vi "GetLastLogFile.vi"(8 "error in (no error)":errorcluster) -> (0 "error out":errorcluster, 2 "Last log file name":string, 3 "Last log file path":path)   [LabVIEW 2013, in "ErrorMessage.lvclass"]
uses:
  001 - MAIN/Class/Messages/ErrorMessage/ErrorMessage.lvclass
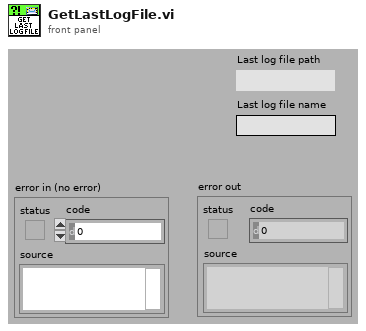
[diagram p1: front panel]
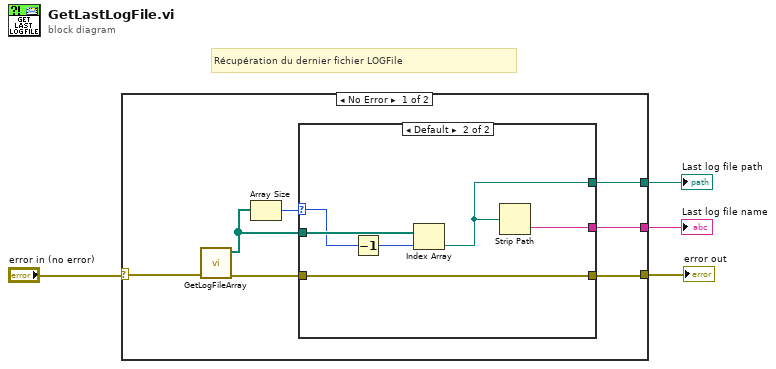
[diagram p0: block diagram]
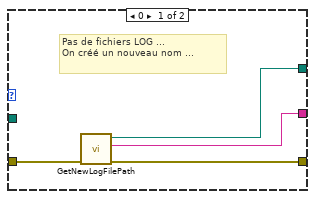
[diagram p2: hidden frame]
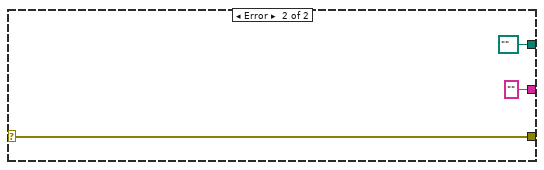
[diagram p3: hidden frame]
diagram:
  # "Récupération du dernier fichier LOGFile"
  n1 = case shown="No Error" "error in (no error)" {
    selector: "error in (no error)" -> [w11 w24]
    tunnel: [w8 "" ("name")] -> w3
    tunnel: [w7 path "" ("Current log file path")] -> w2
    tunnel: [w5 w24] -> w1
    frame No Error {
      n2 = call "GetLogFileArray.vi"("error in (no error)"=w11) -> ("error out"=w9:errorcluster, "LogFileArray"=w6:path[])  [unwired: 8 in, 1 out]
      n3 = Array Size(array=w6) -> (size(s)=w10:i32)
      n4 = case shown="Default" w10 {
        selector: w10 -> [_ w20]
        tunnel: w9 -> [w15 w18]
        tunnel: [w14 w18] -> w5
        tunnel: [w13 w16] -> w8
        tunnel: [w12 w17] -> w7
        tunnel: w6 -> [_ w21]
        frame 0 {
          # "Pas de fichiers LOG ...\nOn créé un nouveau nom ..."
          n5 = call "GetNewLogFilePath.vi"("error in (no error)"=w15) -> ("error out"=w14:errorcluster, "New log filename"=w13:string, "New log file path"=w12:path)  [unwired: 8 in]
        }
        frame Default {
          n6 = Decrement(x=w20) -> (x-1=w19:i32)
          n7 = Index Array(array=w21, index=w19) -> (element=w17:path)
          n8 = Strip Path(path=w17) -> (name=w16:string)  [unwired: 1 out]
        }
      }
    }
    frame Error {
    }
  }
  "error out" <- w1
  "Last log file path" <- w2
  "Last log file name" <- w3
